vi "Get_No_Top_Level_Message.vi"(11 "Build in":refnum<class "AB_Build.lvclass">) -> (2 "No top level VI":string, 3 "Build out":refnum<class "AB_Build.lvclass">)   [LabVIEW 2020, in "AB_Build.lvclass"]
uses:
  <vilib>/AppBuilder/AB_Classes/Build/AB_Build.lvclass
  <vilib>/AppBuilder/AB_Classes/Build/AB_Build.lvclass/AB_Build.ctl
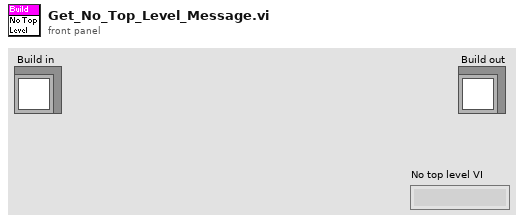
[diagram p1: front panel]
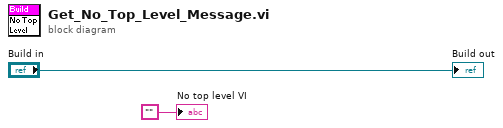
[diagram p0: block diagram]
diagram:
  "No top level VI" <- ""
  "Build out" <- "Build in"
